vi "Enqueue Message Synchron.vi"(6 "Priority Message? (F)":bool, 7 "Notifier":refnum<notifier>, 8 "error in (no error)":errorcluster, 9 "Message Data":variant, 10 "Message":string, 11 "Message Queue":refnum<queue>) -> (0 "error out":errorcluster, 3 "dup Message Queue":refnum<queue>)   [LabVIEW 2017, in "Message Queue.lvlib"]
doc: "For a regular message, enqueue the message. For a priority message, enqueue it at the front of the queue."
uses:
  Message Queue.lvlib
  Message Cluster.ctl
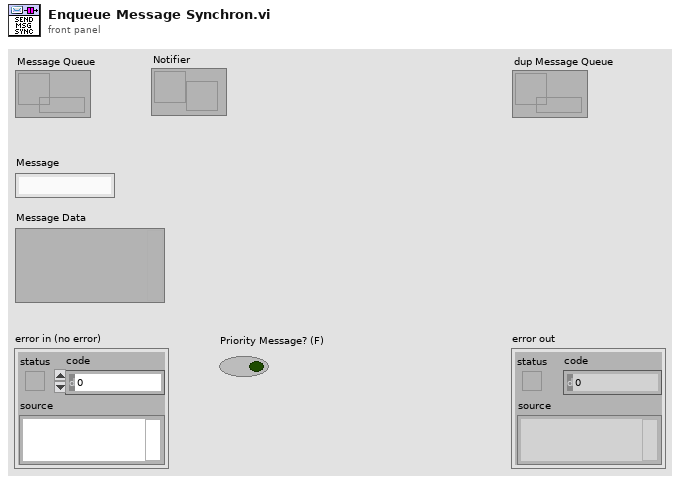
[diagram p1: front panel]
types:
  T1 = typedef "Message Queue.lvlib/Message Cluster.ctl" = cluster{"Message":string, "Message Data":variant}
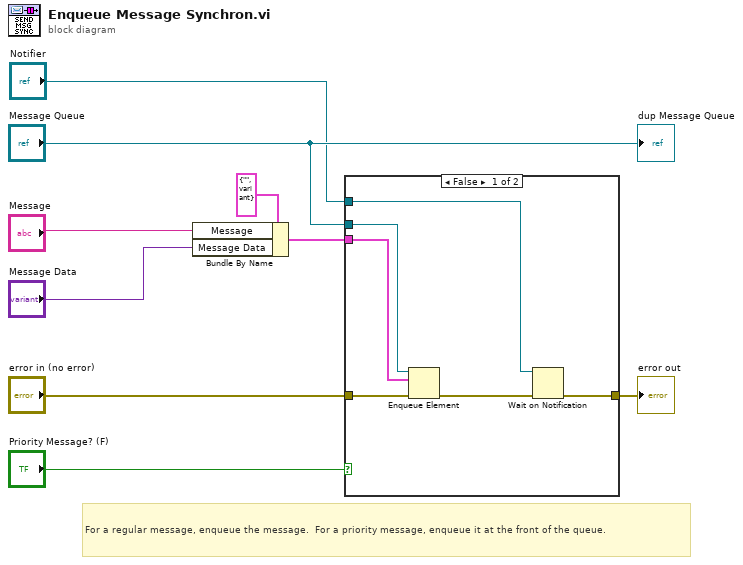
[diagram p0: block diagram]
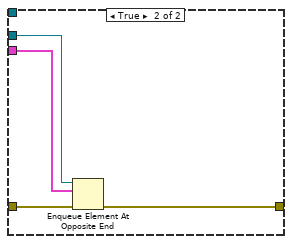
[diagram p2: hidden frame]
diagram:
  # "For a regular message, enqueue the message.  For a priority message, enqueue it at the front of the queue."
  n1 = Bundle By Name(cluster=T1 {"Message"="", "Message Data"=variant} ("Message Cluster"), "Message"="Message", "Message Data"="Message Data") -> (w2:T1)
  n2 = case shown="False" "Priority Message? (F)" {
    tunnel: "error in (no error)" -> [w15 w19]
    tunnel: [w11 w18] -> w4
    tunnel: "Message Queue" -> [w14 w17]
    tunnel: w2 -> [w13 w16]
    tunnel: "Notifier" -> [w10 _]
    frame False {
      n3 = Enqueue Element(queue=w14, element=w13, error in (no error)=w15) -> (error out=w12:errorcluster)  [unwired: 1 in, 2 out]
      n4 = Wait on Notification(notifier=w10, error in (no error)=w12) -> (error out=w11:errorcluster)  [unwired: 2 in, 3 out]
    }
    frame True {
      n5 = Enqueue Element At Opposite End(queue=w17, element=w16, error in (no error)=w19) -> (error out=w18:errorcluster)  [unwired: 1 in, 2 out]
    }
  }
  "error out" <- w4
  "dup Message Queue" <- "Message Queue"
